vi "Logout.vi"(4 "Source (\"\")":string, 8 "error in (no error)":errorcluster, 11 "VISA resource name":refnum<visa-resource-name>) -> (0 "error out":errorcluster, 3 "VISA resource name out":refnum<visa-resource-name>)   [LabVIEW 2011, in "Yokogawa DX Series.lvlib"]
doc: "This VI logouts from the instrument. Then it can not re-login."
uses:
  <instrlib>/Yokogawa DX Series/Yokogawa DX Series.lvlib
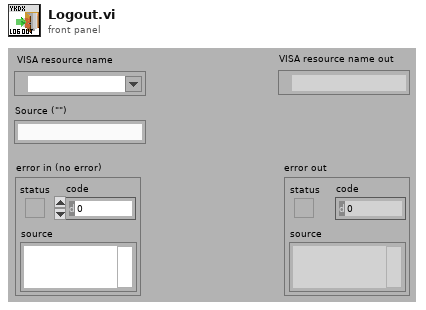
[diagram p1: front panel]
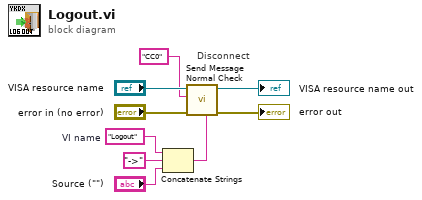
[diagram p0: block diagram]
diagram:
  w9 = "Logout"  # VI name
  # "Disconnect"
  n1 = Concatenate Strings(w9, "->", "Source (\"\")") -> (w3:string)
  n2 = call <instrlib>:"Send Message Normal Check.vi"("Source (\"\")"=w3, "error in (no error)"="error in (no error)", "Send Message (\"\")"="CC0", "VISA resource name"="VISA resource name") -> ("error out"=→"error out":errorcluster, "VISA resource name out"=→"VISA resource name out":refnum<visa-resource-name>)  [unwired: 1 in, 5 out]
